vi "niDAQmx Detach gRPC Task.vi"(0 "task in":refnum<class "Session Factory.lvclass">, 11 "error in":errorcluster) -> (15 "error out":errorcluster)   [LabVIEW 2021, in "Session Management niDAQmx.lvlib" / "Session Factory.lvclass"]
doc: "Detaches from an existing niDAQmx task on the specified NI gRPC Device Server."
uses:
  Session Factory.lvclass
  Session Factory.lvclass/Session Factory.ctl
  NI DAQmx Client/NI_DAQmx_client.lvlib
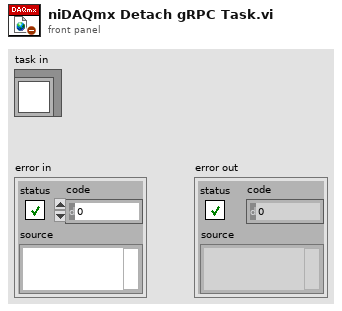
[diagram p1: front panel]
types:
  T1 = typedef "grpc-lvsupport-release.lvlib/grpcId.ctl" = u64
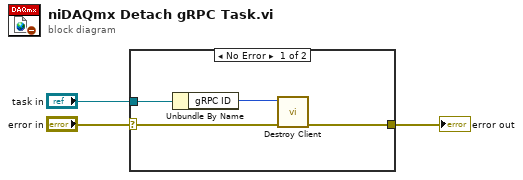
[diagram p0: block diagram]
diagram:
  n1 = case shown="No Error" "error in" {
    selector: "error in" -> [w6 w8]
    tunnel: "task in" -> [w7 _]
    tunnel: [w4 w8] -> w1
    frame No Error {
      n2 = Unbundle By Name(w7) -> ("gRPC ID"=w5:T1)
      n3 = call "Destroy Client.vi"("error in"=w6, "gRPC ID"=w5) -> ("error out"=w4:errorcluster)  [unwired: 9 in]
    }
    frame Error {
    }
  }
  "error out" <- w1
